vi "prime.vi"() -> ()   [LabVIEW 2017]
panel:
  out "COMPOSITE NUMBERS":i32[](array[numeric])
  out "ODD NUMBERS":i32[](array[numeric])
  out "EVEN NUMBERS":i32[](array[numeric])
  out "PRIME NUMBERS":i32[](array[numeric])
  in  "ENTER THE NUMBER":i32
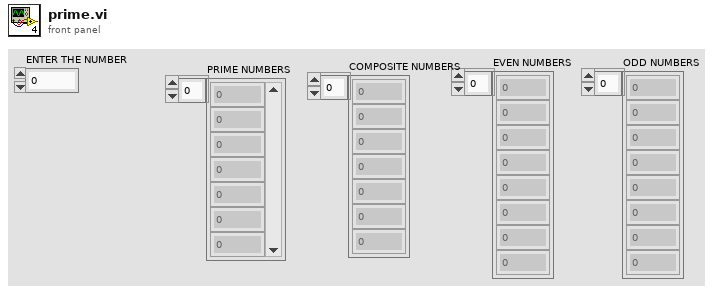
[diagram p1: front panel]
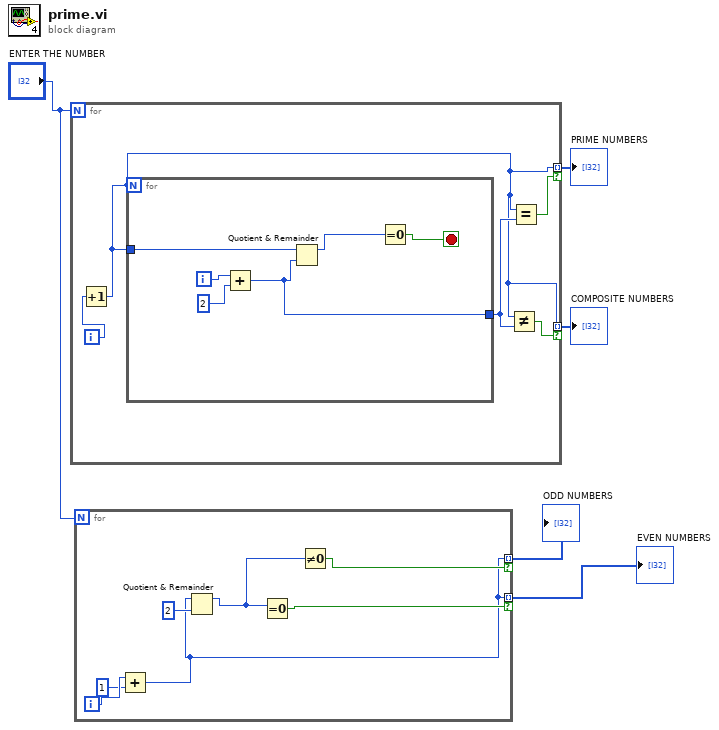
[diagram p0: block diagram]
diagram:
  n1 = for {
    N: "ENTER THE NUMBER" -> [_]
    tunnel: [w6] -> w5 mode=indexing if=w10
    tunnel: [w6] -> w1 mode=indexing if=w8
    i -> [w7]
    n2 = Increment(x=w7) -> (x+1=w6:i32)
    n3 = for {
      N: w6 -> [_]
      tunnel: w6 -> [w14]
      tunnel: [w11] -> w9
      i -> [w16]
      stop <- w12 stop-if-true
      n4 = Add(x=w16, y=2 ("x")) -> (x+y=w11:i32)
      n5 = Quotient & Remainder(x=w14, y=w11) -> (x-y*floor(x/y)=w13:i32)  [unwired: 1 out]
      n6 = Equal To 0?(x=w13) -> (x = 0?=w12:bool)
    }
    n7 = Not Equal?(x=w6, y=w9) -> (x != y?=w8:bool)
    n8 = Equal?(x=w6, y=w9) -> (x = y?=w10:bool)
  }
  "PRIME NUMBERS" <- w5
  "COMPOSITE NUMBERS" <- w1
  n9 = for {
    N: "ENTER THE NUMBER" -> [_]
    tunnel: [w17] -> w3 mode=indexing if=w22
    tunnel: [w17] -> w2 mode=indexing if=w20
    i -> [w19]
    n10 = Add(x=w19, y=1) -> (x+y=w17:i32)
    n11 = Quotient & Remainder(x=w17, y=2) -> (x-y*floor(x/y)=w21:i32)  [unwired: 1 out]
    n12 = Equal To 0?(x=w21) -> (x = 0?=w22:bool)
    n13 = Not Equal To 0?(x=w21) -> (x != 0?=w20:bool)
  }
  "EVEN NUMBERS" <- w3
  "ODD NUMBERS" <- w2
